vi "ConfigureAdditionalProperties.vi"(8 "error in (no error)":errorcluster, 9 "Channels":T1[](array[typedef]), 10 "Channel Properties":T2[](array[typedef]), 11 "Virtual Channel in":T4) -> (0 "error out":errorcluster, 3 "Virtual Channel out":T4)   [LabVIEW 2017, in "McsaVirtualChannel.lvlib"]
uses:
  <vilib>/addons/InsightCM/Devices/Shared/Mcsa/McsaVirtualChannel/McsaVirtualChannel.lvlib
  <vilib>/addons/InsightCM/Devices/Shared/Mcsa/McsaVirtualChannel/controls/VirtualChannel.ctl
  <vilib>/addons/InsightCM/MessageBus/Base/controls/KeyValuePair.ctl
  <vilib>/addons/InsightCM/MessageBus/Base/controls/R2_Channel.ctl
  <vilib>/addons/InsightCM/MessageBus/Base/controls/Metric.ctl
  <vilib>/addons/InsightCM/Utilities/Analysis/MCSA/McsaAnalysisFunctions.lvlib
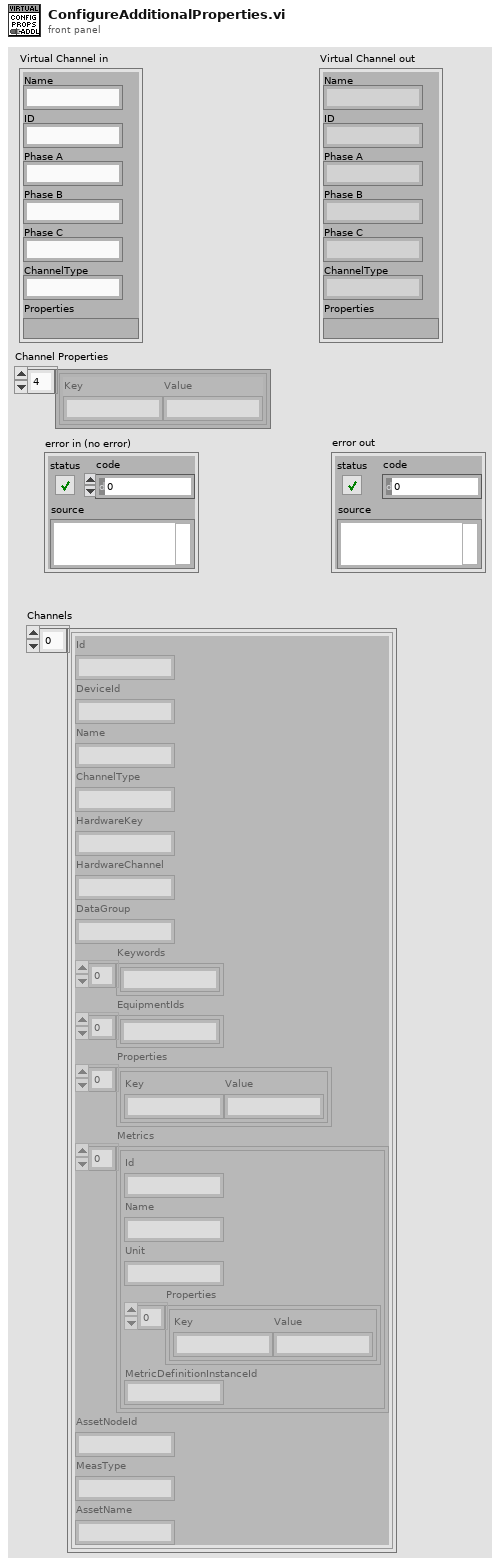
[diagram p1: front panel]
types:
  T1 = typedef "R2_Channel.ctl" = cluster{"Id":string, "DeviceId":string, "Name":string, "ChannelType":string, "HardwareKey":string, "HardwareChannel":string, "DataGroup":string, "Keywords":string[], "EquipmentIds":string[], "Properties":T2[], "Metrics":T3[], "AssetNodeId":string, "MeasType":string, "AssetName":string}
  T2 = typedef "KeyValuePair.ctl" = cluster{"Key":string, "Value":string}
  T3 = typedef "Metric.ctl" = cluster{"Id":string, "Name":string, "Unit":string, "Properties":T2[], "MetricDefinitionInstanceId":string}
  T4 = typedef "McsaVirtualChannel.lvlib/VirtualChannel.ctl" = cluster{"Name":string, "ID":string, "Phase A":string, "Phase B":string, "Phase C":string, "ChannelType":string, "Properties":variant}
  T5 = typedef "McsaVirtualChannel.lvlib/VoltageBus.ctl" = cluster{"Wiring Configuration":string, "Nominal Voltage":dbl}
  T6 = typedef "McsaAnalysisFunctions.lvlib/McsaMotor.ctl" = cluster{"Model":string, "Manufacturer":string, "Serial Number":string, "Horsepower":dbl, "Horsepower Unit":string, "Full Load Speed":dbl, "Synchronous Speed":dbl, "Rated Volts":dbl, "Full Load Amps":dbl, "Frequency":dbl, "Service Factor":dbl, "Efficiency":dbl, "Efficiency @ 75% Load":dbl, "Efficiency @ 50% Load":dbl, "Efficiency @ 25% Load":dbl, "Power Factor":dbl, "VoltageBus":string, "VoltageBus ID":string, "Stator Resistance":dbl, "Estimate Stator Resistance":bool}
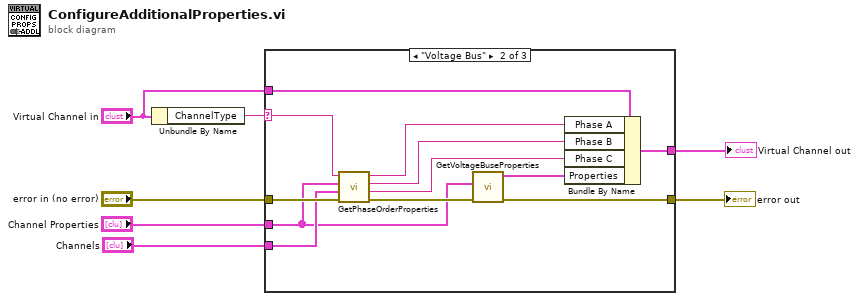
[diagram p0: block diagram]
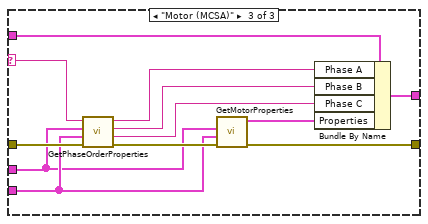
[diagram p3: hidden frame]
diagram:
  n1 = Unbundle By Name("Virtual Channel in") -> ("ChannelType"=w7:string)
  n2 = case shown="\"Voltage Bus\"" w7 {
    selector: w7 -> [_ w10 w22]
    tunnel: [w8 w20 w32] -> w1
    tunnel: "Virtual Channel in" -> [w8 w21 w33]
    tunnel: "error in (no error)" -> [w9 w16 w28]
    tunnel: [w9 w19 w31] -> w3
    tunnel: "Channel Properties" -> [_ w11 w23]
    tunnel: "Channels" -> [_ w15 w27]
    frame Default {
    }
    frame "Voltage Bus" {
      n3 = call <vilib>:"GetPhaseOrderProperties.vi"("error in (no error)"=w16, "Channels"=w15, "Channel Properties"=w11, "ChannelType"=w10) -> ("error out"=w17:errorcluster, "Phase C ChannelName"=w13:string, "Phase B ChannelName"=w14:string, "Phase A ChannelName"=w12:string)  [unwired: 3 in, 1 out]
      n4 = call <vilib>:"GetVoltageBuseProperties.vi"("error in (no error)"=w17, "Channel Properties"=w11) -> ("error out"=w19:errorcluster, "VoltageBus"=w18:T5)  [unwired: 8 in]
      n5 = Bundle By Name(cluster=w21, "Phase A"=w12, "Phase B"=w14, "Phase C"=w13, "Properties"=w18) -> (w20:T4)
    }
    frame "Motor (MCSA)" {
      n6 = call <vilib>:"GetPhaseOrderProperties.vi"("error in (no error)"=w28, "Channels"=w27, "Channel Properties"=w23, "ChannelType"=w22) -> ("error out"=w29:errorcluster, "Phase C ChannelName"=w25:string, "Phase B ChannelName"=w26:string, "Phase A ChannelName"=w24:string)  [unwired: 3 in, 1 out]
      n7 = call <vilib>:"GetMotorProperties.vi"("error in (no error)"=w29, "Channels"=w27, "Channel Properties"=w23) -> ("error out"=w31:errorcluster, "Motor"=w30:T6)  [unwired: 6 in, 1 out]
      n8 = Bundle By Name(cluster=w33, "Phase A"=w24, "Phase B"=w26, "Phase C"=w25, "Properties"=w30) -> (w32:T4)
    }
  }
  "Virtual Channel out" <- w1
  "error out" <- w3
